vi "Actor Core.vi"(8 "error in":errorcluster, 11 "Generator in":refnum<class "Generator.lvclass">) -> (0 "error out":errorcluster, 3 "Actor out":refnum<class "Actor.lvclass">)   [LabVIEW 2020, in "Wrapped Actor.lvlib" / "Generator.lvclass"]
doc: "(<B>Filename</B>: Actor Framework.lvlib:Actor.lvclass:Actor Core.vi)\n\nReceives messages to the actor, reacts to them, and initiates any error handling that may shut the actor down.\n\nDescendant classes may override this VI to append parallel tasks for the actor to complete while it handles messages. Overrides use the Call Parent Class Method node."
uses:
  Generator.lvclass
  <vilib>/ActorFramework/Actor/Actor.lvclass
  Generator.lvclass/Generator.ctl
  <vilib>/MGI/Monitored Actor/Monitored Actor/Monitored Actor/Monitored Actor.lvclass
  Data Message/Data Message.lvclass
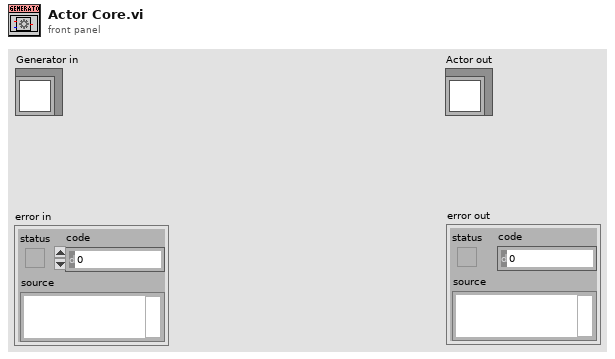
[diagram p1: front panel]
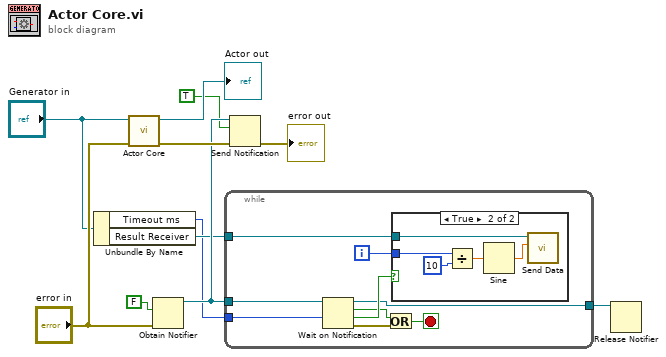
[diagram p0: block diagram]
diagram:
  n1 = Unbundle By Name("Generator in") -> ("Timeout ms"=w1:i32, "Result Receiver"=w4:refnum<class "Message Enqueuer.lvclass">)
  n2 = call-parent "Actor Core.vi"("error in"="error in", "Actor in"="Generator in") -> ("error out"=w8:errorcluster, "Actor out"=→"Actor out":refnum<class "Actor.lvclass">)  [unwired: 8 in]
  n3 = Obtain Notifier(notification data type=FALSE, error in (no error)="error in") -> (notifier out=w7:refnum<notifier>)  [unwired: 2 in, 2 out]
  n4 = while {
    tunnel: w7 -> [w20]
    tunnel: w4 -> [w15]
    tunnel: [w13] -> w2
    tunnel: w1 -> [w12]
    i -> [w14]
    stop <- w17 stop-if-true
    n5 = Wait on Notification(notifier=w20, timeout in ms (-1)=w12) -> (notifier out=w13:refnum<notifier>, notification=w18:bool, timed out?=w19:bool, error out=w16:errorcluster)  [unwired: 2 in]
    n6 = Or(x=w18, y=w16) -> (x .or. y?=w17:bool)
    n7 = case shown="True" w19 {
      tunnel: w15 -> [_ w25]
      tunnel: w14 -> [_ w24]
      frame False {
      }
      frame True {
        n8 = Divide(x=w24, y=10) -> (x/y=w23:dbl)
        n9 = Sine(x=w23) -> (sin(x)=w21:dbl)
        n10 = call "Send Data.vi"("Value"=w21, "Destination"=w25) -> ()  [unwired: 9 in, 1 out]
      }
    }
  }
  n11 = Send Notification(notification=TRUE, notifier=w7, error in (no error)=w8) -> (error out=→"error out":errorcluster)  [unwired: 1 out]
  n12 = Release Notifier(notifier=w2) -> ()  [unwired: 2 in, 3 out]
